vi "soft_control.vi"(4 "手动输入":dbl, 7 "开始控制":bool, 8 "PID gains":T1={"proportional gain (Kc)"=43.0, "integral time (Ti, min)"=0.1, "derivative time (Td, min)"=0.0001} caption="PID增益" {"derivative time (Td, min)" format="%.6f"; "integral time (Ti, min)" format="%.7f"; "proportional gain (Kc)" format="%.3f"}, 9 "reinitialize? (F)":bool=TRUE caption="重新初始化？(F)", 10 "启用自动输入":bool) -> (0 "实际弯曲角":dbl, 1 "PID输出":dbl, 2 "误差":dbl, 3 "理想弯曲角":dbl, 5 "速度输入":dbl)   [LabVIEW 2020]
uses:
  <vilib>/Platform/TimedLoop/XDataNode/wakeup.ctl
  <vilib>/Platform/TimedLoop/XDataNode/XDNodeRunTimeDep.lvlib
  <vilib>/Platform/TimedLoop/XDataNode/nitl_modes.ctl
  <vilib>/Platform/TimedLoop/XDataNode/timing_clust.ctl
  <vilib>/Platform/TimedLoop/XDataNode/XDataNode.xnode
  <vilib>/addons/control/pid/NI_PID_pid.lvlib
  <vilib>/imath/engines/lvmath2/RunTimeEngine/BuiltInFunctions/mod/NIMS_mod_no_size_check.vi
  <vilib>/imath/engines/lvmath2/RunTimeEngine/NodeEndStatement/NIMS_NodeEndStatement_Output.vi
  <vilib>/imath/engines/lvmath2/RunTimeEngine/ErrorHandling/NIMS_Finalize Error.vi
  <vilib>/addons/control/pid/pid.llb/PID (DBL).vi
panel:
  out "valve6Switch":bool=TRUE
  out "valve5Switch":bool
  out "valve4Switch":bool=TRUE
  out "valve3Switch":bool
  out "valve2Switch":bool
  out "valve1Switch":bool
  out "时间":dbl=73.22
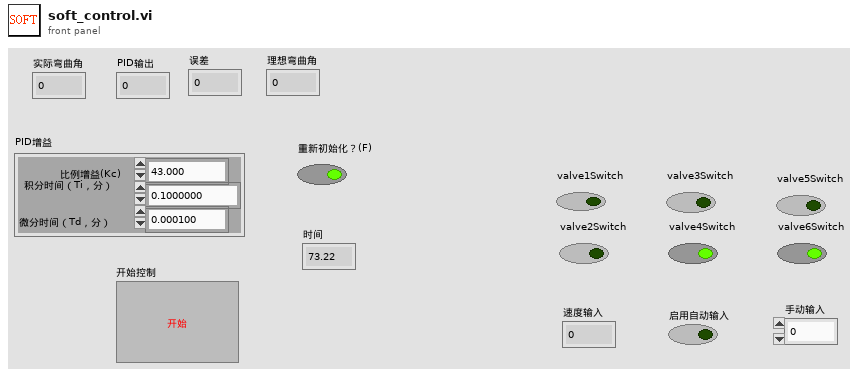
[diagram p1: front panel]
types:
  T1 = cluster{"proportional gain (Kc)":dbl, "integral time (Ti, min)":dbl, "derivative time (Td, min)":dbl}
  T2 = typedef "XDNodeRunTimeDep.lvlib/timing_clust.ctl" = cluster{"Expected End [f-1]":u64, "Actual End [f-1]":u64, "Finished Late? [f-1]":bool, "Expected End [i-1]":u64, "Actual End [i-1]":u64, "Finished Late? [i-1]":bool, "Expected Start [i]":u64, "Actual Start [i]":u64, "Expected Start [f]":u64, "Actual Start [f]":u64, "Source Name":string, "Structure Name":string, "Period":i64, "Deadline":i64, "Offset":i64, "Start":i64, "Priority":i32, "Timeout":i32, "Mode":T3, "Wakeup Reason":T4, "Error":errorcluster, "Source Type":string, "Secondary Source Type":string, "Global End Time":u64, "Global Start Time":u64, "Frame Duration":u64, "Iteration Duration":u64, "Assigned CPU":i32, "I/O Scan Engine Mode":u32}
  T3 = typedef "XDNodeRunTimeDep.lvlib/nitl_modes.ctl" = enum32{"No Change", "Process missed periods, maintain original phase", "Discard missed periods, maintain original phase", "Process missed periods, ignore original phase", "Discard missed periods, ignore original phase"}
  T4 = typedef "XDNodeRunTimeDep.lvlib/wakeup.ctl" = enum32{"Normal", "Aborted", "Asynchronous wakeup", "Timing source error", "Timed loop error", "Timeout"}
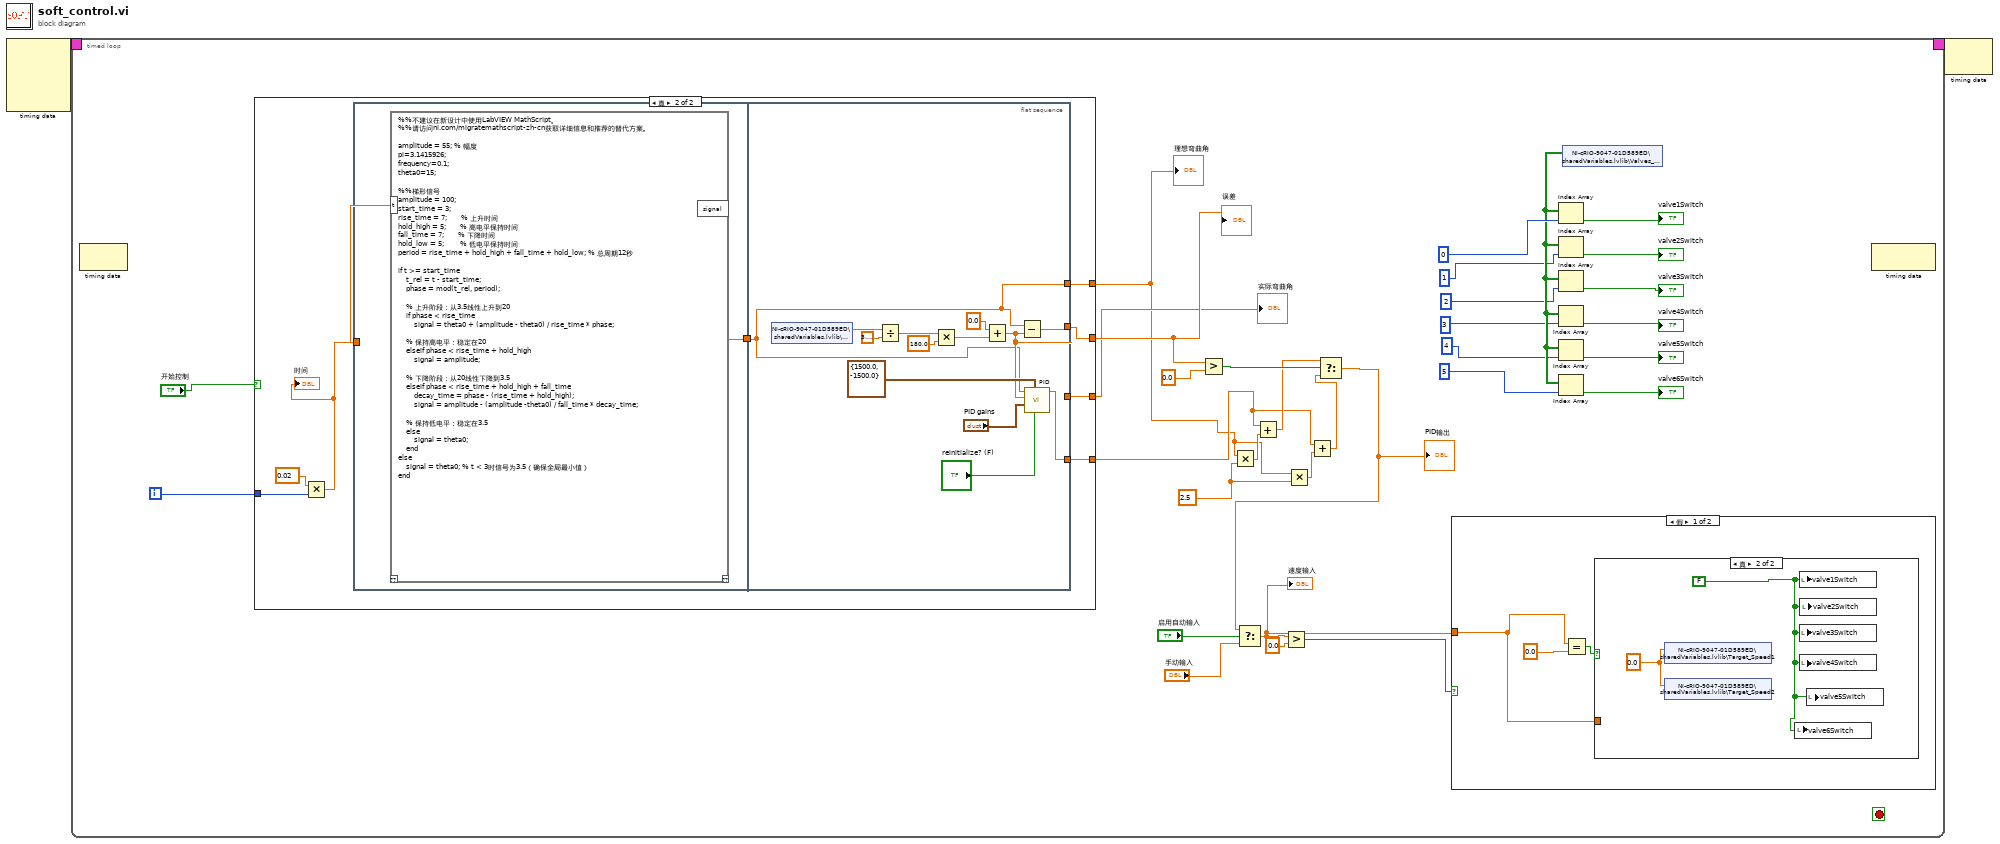
[diagram p0: block diagram]
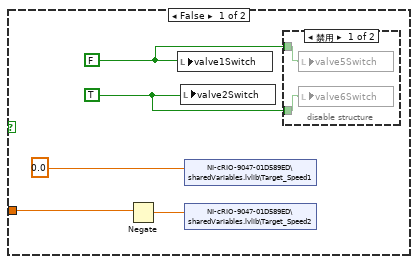
[diagram p2: hidden frame]
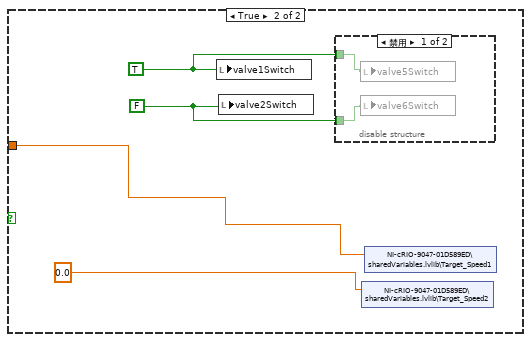
[diagram p4: hidden frame]
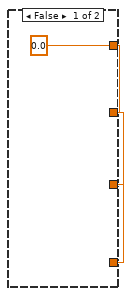
[diagram p6: hidden frame]
diagram:
  n1 = node-c288() -> (w2:T2)  [unwired: 4 in]
  n2 = timed-loop {
    timing: w2 -> [_]
    timing-out: [_] -> w1
    i -> [w33]
    stop <- _ stop-if-true
    w9 = 2.5 ("y")
    n3 = node-c288() -> ()  [unwired: 1 in, 1 out]
    n4 = case shown="真" "开始控制" {
      tunnel: w33 -> [_ w58]
      tunnel: [w53 w54] -> w3
      tunnel: [w53 w57] -> w6
      tunnel: [w53 w56] -> w5
      tunnel: [w53 w55] -> w7
      frame False {
        w53 = 0.0 ("signal")
      }
      frame True {
        n5 = Multiply(x=0.02, y=w58) -> (x*y=w59:dbl)
        "时间" <- w59
        n6 = flat-sequence {
          tunnel: w59 -> [w63]
          tunnel: [w62] -> w61
          tunnel: w61 -> [w290]
          tunnel: [w290] -> w54
          tunnel: [w293] -> w57
          tunnel: [w292] -> w56
          tunnel: [w291] -> w55
          frame #0 {
            n7 = mathscript code="%%不建议在新设计中使用LabVIEW MathScript。\n%%请访问ni.com/migratemathscript-zh-cn获取详细信息和推荐的替代方案。\n\namplitude = 55; % 幅度\npi=3.1415926;\nfrequency=0.1;\ntheta0=15;\n\n%%梯形信号\namplitude = 100;\nstart_time = 3;\nrise_time = 7;       % 上升时间\nhold_high = 5;       % 高电平保持时间\nfall_time = 7;       % 下降时间\nhold_low = 5;        % 低电平保持时间\nperiod = rise_time + hold_high + fall_time + hold_low; % 总周期12秒\n\nif t >= start_time\n    t_rel = t - start_time;\n    phase = mod(t_rel, period);\n    \n    % 上升阶段：从3.5线性上升到20\n    if phase < rise_time\n        signal = theta0 + (amplitude - theta0) / rise_time * phase;\n    \n    % 保持高电平：稳定在20\n    elseif phase < rise_time + hold_high\n        signal = amplitude;\n    \n    % 下降阶段：从20线性下降到3.5\n    elseif phase < rise_time + hold_high + fall_time\n        decay_time = phase - (rise_time + hold_high);\n        signal = amplitude - (amplitude -theta0) / fall_time * decay_time;\n    \n    % 保持低电平：稳定在3.5\n    else\n        signal = theta0;\n    end\nelse\n    signal = theta0; % t < 3时信号为3.5（确保全局最小值）\nend"("t"=w63) -> ("signal"=w62:dbl)  [unwired: 1 in, 1 out]
          }
          frame #1 {
            n8 = shared-variable "NI-cRIO-9047-01D589ED\\sharedVariables.lvlib\\armTheta"() -> (w300:dbl)  [unwired: 1 in, 1 out]
            n9 = Divide(x=w300, y=3.141592653589793) -> (x/y=w298:dbl)
            n10 = Multiply(x=w298, y=180.0) -> (x*y=w295:dbl)
            n11 = Add(x=0.0, y=w295) -> (x+y=w292:dbl)
            n12 = Subtract(x=w290, y=w292) -> (x-y=w293:dbl)
            n13 = call-poly <vilib>:"PID.vi"("reinitialize? (F)"="reinitialize? (F)", "output range"=cluster{"output high":dbl, "output low":dbl} {"output high"=1500.0, "output low"=-1500.0}, "PID gains"="PID gains", "process variable"=w292, "setpoint"=w290) -> ("output"=w291:dbl)  [unwired: 5 in, 1 out]
          }
        }
      }
    }
    "误差" <- w6
    "理想弯曲角" <- w3
    "实际弯曲角" <- w5
    n14 = Greater?(x=w6, y=0.0) -> (0:w12:bool)
    n15 = Multiply(x=w3, y=w9) -> (x*y=w14:dbl)
    n16 = Add(x=w7, y=w14) -> (x+y=w11:dbl)
    n17 = Multiply(x=w3, y=w9) -> (x*y=w10:dbl)
    n18 = Add(x=w7, y=w10) -> (x+y=w8:dbl)
    n19 = Select(t=w11, s=w12, f=w8) -> (s? t:f=w4:dbl)
    "PID输出" <- w4
    n20 = Select(t=w4, s="启用自动输入", f="手动输入") -> (s? t:f=w32:dbl)
    "速度输入" <- w32
    n21 = Greater?(x=w32, y=0.0) -> (0:w31:bool)
    n22 = case shown="假" w31 {
      tunnel: w32 -> [w35 w48]
      frame False {
        n23 = Equal?(x=w35, y=0.0) -> (x = y?=w36:bool)
        n24 = case shown="真" w36 {
          tunnel: w35 -> [w40 _]
          frame False {
            w42 = FALSE
            w41 = TRUE
            n25 = Negate(x=w40) -> (-x=w39:dbl)
            n26 = local write "valve1Switch"(w42) -> ()
            n27 = local write "valve2Switch"(w41) -> ()
            n28 = shared-variable "NI-cRIO-9047-01D589ED\\sharedVariables.lvlib\\Target_Speed1"(0.0 ("目标速度  1")) -> ()  [unwired: 1 in, 1 out]
            n29 = shared-variable "NI-cRIO-9047-01D589ED\\sharedVariables.lvlib\\Target_Speed2"(w39) -> ()  [unwired: 1 in, 1 out]
            n30 = disable-structure shown="禁用" {
              disable-tunnel: w42 -> [w44 _]
              disable-tunnel: w41 -> [w43 _]
              frame Disabled {
                n31 = local write "valve5Switch"(w44) -> ()
                n32 = local write "valve6Switch"(w43) -> ()
              }
              frame Enabled {
              }
            }
          }
          frame True {
            w45 = 0.0 ("y")
            w46 = FALSE ("valve1Switch")
            n33 = shared-variable "NI-cRIO-9047-01D589ED\\sharedVariables.lvlib\\Target_Speed1"(w45) -> ()  [unwired: 1 in, 1 out]
            n34 = shared-variable "NI-cRIO-9047-01D589ED\\sharedVariables.lvlib\\Target_Speed2"(w45) -> ()  [unwired: 1 in, 1 out]
            n35 = local write "valve6Switch"(w46) -> ()
            n36 = local write "valve1Switch"(w46) -> ()
            n37 = local write "valve3Switch"(w46) -> ()
            n38 = local write "valve4Switch"(w46) -> ()
            n39 = local write "valve2Switch"(w46) -> ()
            n40 = local write "valve5Switch"(w46) -> ()
          }
        }
      }
      frame True {
        w49 = FALSE
        w50 = TRUE
        n41 = local write "valve1Switch"(w50) -> ()
        n42 = local write "valve2Switch"(w49) -> ()
        n43 = disable-structure shown="禁用" {
          disable-tunnel: w50 -> [w52 _]
          disable-tunnel: w49 -> [w51 _]
          frame Disabled {
            n44 = local write "valve5Switch"(w52) -> ()
            n45 = local write "valve6Switch"(w51) -> ()
          }
          frame Enabled {
          }
        }
        n46 = shared-variable "NI-cRIO-9047-01D589ED\\sharedVariables.lvlib\\Target_Speed2"(0.0) -> ()  [unwired: 1 in, 1 out]
        n47 = shared-variable "NI-cRIO-9047-01D589ED\\sharedVariables.lvlib\\Target_Speed1"(w48) -> ()  [unwired: 1 in, 1 out]
      }
    }
    n48 = shared-variable "NI-cRIO-9047-01D589ED\\sharedVariables.lvlib\\Valves_Switch"() -> (w25:bool[])  [unwired: 1 in, 1 out]
    n49 = Index Array(array=w25, index=0) -> (element=→"valve1Switch":bool)
    n50 = Index Array(array=w25, index=1) -> (element=→"valve2Switch":bool)
    n51 = Index Array(array=w25, index=2) -> (element=→"valve3Switch":bool)
    n52 = Index Array(array=w25, index=3) -> (element=→"valve4Switch":bool)
    n53 = Index Array(array=w25, index=4) -> (element=→"valve5Switch":bool)
    n54 = Index Array(array=w25, index=5) -> (element=→"valve6Switch":bool)
    n55 = node-c288() -> ()  [unwired: 1 in, 1 out]
  }
  n56 = node-c288(w1) -> ()  [unwired: 1 out]
